vi "MSGR Group Send.vi"(0 "MSGR Q names":T1[](array[typedef]), 5 "Msg":string, 7 "Reply?":bool, 9 "ReplyQ":string, 11 "error in (no error)":errorcluster, 12 "timeout in ms (-1)":i32=-1) -> (8 "timed out?":bool, 15 "error out":errorcluster)   [LabVIEW 2018]
doc: "$Author::Richard Jennings $\n$Rev:: $\n$Date:: May, 2008 $\n\nOVERVIEW:\nReentrant VI to receive messages via a MSGR Q. If the Q does not exist this VI will create it, then wait for data.\n\nINPUTS (Controls):\n<name> - <short description of each control wired to connector pane>\n\nOUTPUTS (Indicators):\n<name> - <short description of each indicator wired to connector pane>\n\nCopyright 2008 - 2017 Jennings Embedded Servies. All rights reserved.\nAuthor makes no warranties or guarantees related to performance of the software.\nUSE AT YOUR OWN RISK\nwww.jembedded.com"
uses:
  MSGR Q Name TypeDef.ctl
  MSGR Q Data TypeDef.ctl
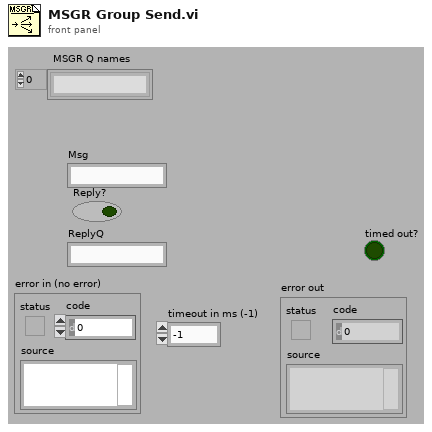
[diagram p1: front panel]
types:
  T1 = typedef "MSGR Q Name TypeDef.ctl" = string
  T2 = typedef "MSGR Q Data TypeDef.ctl" = cluster{"Msg":string, "Parameters":string, "Reply?":bool, "ReplyQ":string}
  T3 = typedef "MSGR Q Ref TypeDef.ctl" = refnum<queue>
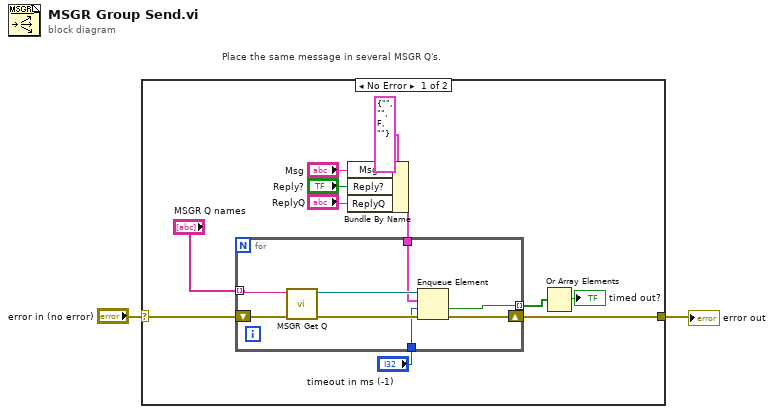
[diagram p0: block diagram]
diagram:
  # "Place the same message in several MSGR Q's."
  n1 = case shown="No Error" "error in (no error)" {
    selector: "error in (no error)" -> [w3 w22]
    tunnel: [w8 w22] -> w2
    frame No Error {
      n2 = Bundle By Name(cluster=T2 {"Msg"="", "Parameters"="", "Reply?"=FALSE, "ReplyQ"=""} ("element"), "Msg"="Msg", "Reply?"="Reply?", "ReplyQ"="ReplyQ") -> (w12:T2)
      n3 = for {
        tunnel: w12 -> [w18]
        shift-right: [w17] -> w8
        shift-left: w3 -> [w21]
        tunnel: "MSGR Q names" -> [w16] mode=indexing
        tunnel: [w15] -> w7 mode=indexing
        tunnel: "timeout in ms (-1)" -> [w14]
        n4 = call "MSGR Get Q.vi"("error in (no error)"=w21, "MSGR Q name"=w16) -> ("error out"=w20:errorcluster, "MSGR Q"=w19:T3)  [unwired: 8 out]
        n5 = Enqueue Element(queue=w19, element=w18, timeout in ms (-1)=w14, error in (no error)=w20) -> (timed out?=w15:bool, error out=w17:errorcluster)  [unwired: 1 out]
      }
      n6 = Or Array Elements(Boolean array=w7) -> (logical OR=→"timed out?":bool)
    }
    frame Error {
    }
  }
  "error out" <- w2
